vi "DSP.vi"(0 "Input Signal":dbl[](array[numeric]), 1 "Smooth(F : Don't)":bool, 2 "Minus Noise(F : Don't)":bool, 5 "RF":T1 {"Forward Coefficients" format="%.4f"; "Reverse Coefficients" format="%.4f"}, 7 "IIR Filter Cluster":T1 caption="IIR滤波器簇" {"Forward Coefficients" format="%.4f"; "Reverse Coefficients" format="%.4f"}, 9 "Noise Signal":dbl[](array[numeric]), 11 "error in (no error)":errorcluster caption="错误输入（无错误）", 12 "SPAN":i32, 13 "Logarithmic Base":dbl) -> (4 "DSP signal":dbl[](array[numeric]), 15 "error out":errorcluster caption="错误输出")   [LabVIEW 2015, in "Digital Signal Processing.lvlib"]
uses:
  Digital Signal Processing.lvlib
  <vilib>/Analysis/baseanly.llb/IIR Cascade Filter (DBL).vi
  <vilib>/Analysis/NI_AALBase.lvlib
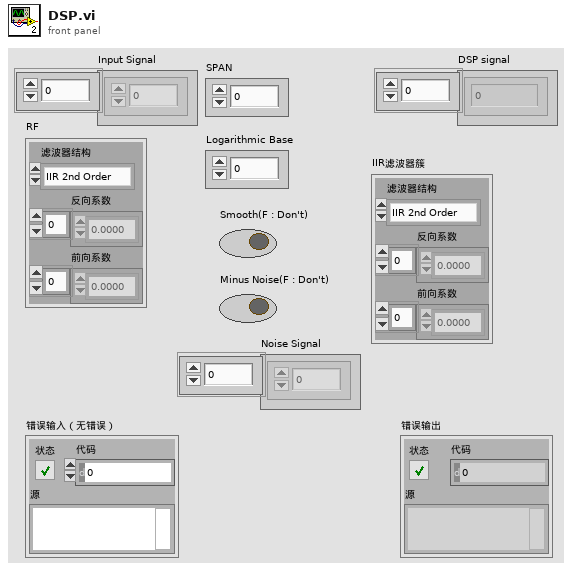
[diagram p1: front panel]
types:
  T1 = cluster{"filter structure":enum32{"IIR 2nd Order", "IIR 4th Order"}, "Reverse Coefficients":dbl[], "Forward Coefficients":dbl[]}
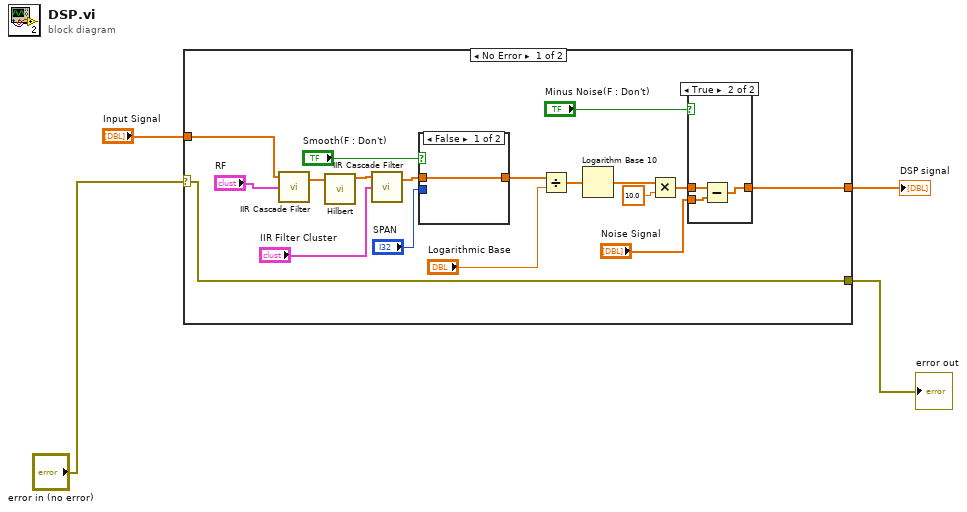
[diagram p0: block diagram]
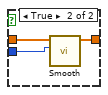
[diagram p2: hidden frame]
diagram:
  n1 = case shown="No Error" "error in (no error)" {
    selector: "error in (no error)" -> [w10 w31]
    tunnel: "Input Signal" -> [w8 _]
    tunnel: [w10 w31] -> w2
    tunnel: [w5 _] -> w1
    frame No Error {
      n2 = call-poly <vilib>:"IIR Cascade Filter.vi"("IIR Filter Cluster"="RF", "X"=w8) -> ("Filtered X"=w7:dbl[])  [unwired: 1 in, 1 out]
      n3 = call "Hilbert.vi"("X"=w7) -> ("H(X)"=w13:dbl[])  [unwired: 10 in]
      n4 = call-poly <vilib>:"IIR Cascade Filter.vi"("IIR Filter Cluster"="IIR Filter Cluster", "X"=w13) -> ("Filtered X"=w12:dbl[])  [unwired: 1 in, 1 out]
      n5 = case shown="False" "Smooth(F : Don't)" {
        tunnel: w12 -> [w23 w26]
        tunnel: "SPAN" -> [_ w25]
        tunnel: [w23 w24] -> w6
        frame False {
        }
        frame True {
          n6 = call "Smooth.vi"("SPAN"=w25, "S"=w26) -> ("S_smooth"=w24:dbl[])  [unwired: 9 in]
        }
      }
      n7 = Divide(x=w6, y="Logarithmic Base") -> (x/y=w22:dbl[])
      n8 = Logarithm Base 10(1:w22) -> (0:w20:dbl[])
      n9 = Multiply(x=w20, y=10.0) -> (x*y=w14:dbl[])
      n10 = case shown="True" "Minus Noise(F : Don't)" {
        tunnel: w14 -> [w27 w30]
        tunnel: "Noise Signal" -> [_ w29]
        tunnel: [w27 w28] -> w5
        frame False {
        }
        frame True {
          n11 = Subtract(x=w30, y=w29) -> (x-y=w28:dbl[])
        }
      }
    }
    frame Error {
    }
  }
  "DSP signal" <- w1
  "error out" <- w2
